vi "write_binary.vi"   [LabVIEW 2021]
types:
  T1 = enum16{"open", "replace", "create", "open or create", "replace or create", "replace or create with confirmation"}
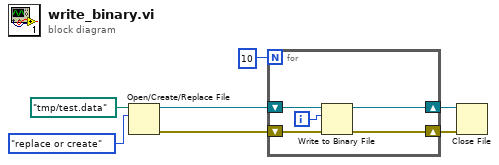
[diagram p0: block diagram]
diagram:
  n1 = Open/Create/Replace File(file path (use dialog)=path "/tmp/test.data", operation (0:open)=T1."replace or create") -> (refnum out=w7:refnum<file>, error out=w6:errorcluster)  [unwired: 4 in, 1 out]
  n2 = for {
    N: 10 -> [_]
    shift-right: [w10] -> w5
    shift-left: w7 -> [w12]
    shift-right: [w9] -> w4
    shift-left: w6 -> [w11]
    i -> [w8]
    n3 = Write to Binary File(file (use dialog)=w12, data=w8, error in=w11) -> (refnum out=w10:refnum<file>, error out=w9:errorcluster)  [unwired: 3 in, 1 out]
  }
  n4 = Close File(refnum=w5, error in=w4) -> ()  [unwired: 2 out]
